vi "Find Multiple Items.vi"(7 "$Path or Item Name":string, 8 "error in (no error)":errorcluster, 10 "Offset":i32, 11 "JSON":string) -> (0 "error out":errorcluster, 1 "<JSON>":string[](array[string]) caption="<JSON>Items", 2 "Item Offsets":i32[](array[numeric]), 3 "Item Names":string[](array[string]))   [LabVIEW 2019, in "JSONtext.lvlib"]
doc: "Find the JSON items at the JSON Path specified and returns them as an array.\n\nPaths specify an item in a tree of nested Elements, and start with $. Each element is either in the form .name, for Object items, or [n] for Array index ([*] for all elements). Multiple Object items can be specified by the list form .[abc,def].\n\nIf the Path input does not start with a $, then it is interpreted as a single Object Item name, rather than a path.\n\nExample JSON:\n{\"A\":[{\"C\":123,\"D\":4},{\"C\":567,\"D\":8}],\"B\":{\"F\":9},\"E\":true}\nAt path $.A[*].C are 123 and 567\nAt path $.B (or just B) is {\"F\":9}\nAt path $.B.F is 9\nAt path $.[B,E] are {\"F\":9} and true"
uses:
  JSONtext.lvlib
  support/Unescape JSON string.vi
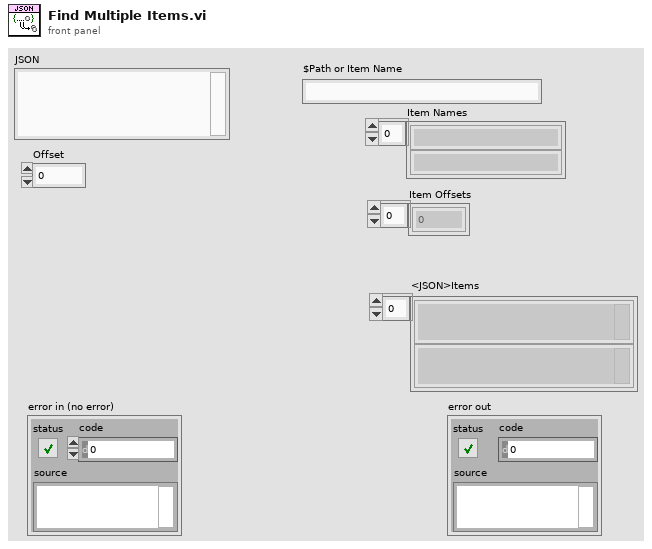
[diagram p1: front panel]
types:
  T1 = typedef "JSONtext.lvlib/Found Items.ctl" = cluster{"Item offset":i32, "Offset past Item":i32, "Name offset":i32, "Offset past Name":i32, "Found":bool, "Item Type":T2, "Item Index":i32, "Start Offset":i32, "Comma Needed For Insert":bool}
  T2 = typedef "JSONtext.lvlib/Parsing State.ctl" = enum16{"Parser Error", "Object", "Array", "String", "Number/Other", "Leading Whitespace", "Object end", "Array end", "Value end"}
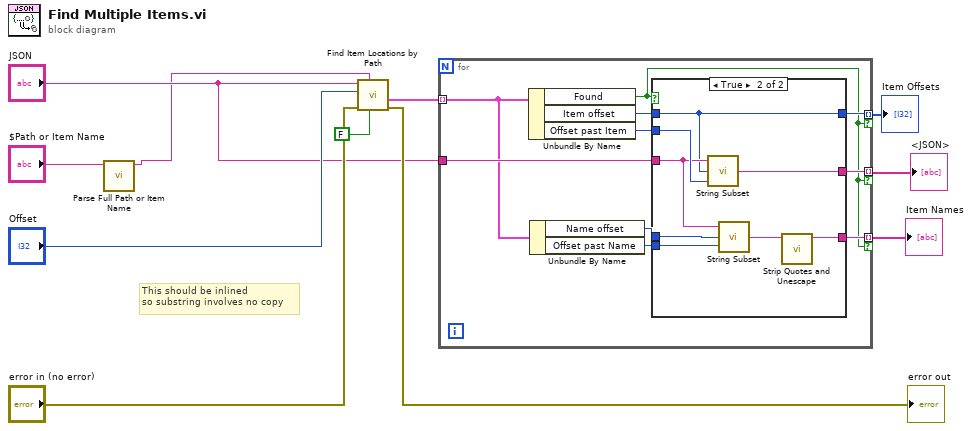
[diagram p0: block diagram]
diagram:
  # "This should be inlined\nso substring involves no copy"
  n1 = call "Parse Full Path or Item Name.vi"("Full Path (with $) or Name"="$Path or Item Name") -> ("Relative Path or JSON-format name"=w1:string)  [unwired: 10 in]
  n2 = call "Find Item Locations by Path.vi"("Only return first found"=FALSE, "Path"=w1, "error in (no error)"="error in (no error)", "Offset"="Offset", "JSON"="JSON") -> ("error out"=→"error out":errorcluster, "Items"=w6:T1[])  [unwired: 5 in]
  n3 = for {
    tunnel: "JSON" -> [w21]
    tunnel: [w20] -> w7 mode=indexing if=w12
    tunnel: w6 -> [w17] mode=indexing
    tunnel: [w14] -> w5 mode=indexing if=w12
    tunnel: [w13] -> w3 mode=indexing if=w12
    n4 = Unbundle By Name(w17) -> ("Found"=w12:bool, "Item offset"=w19:i32, "Offset past Item"=w18:i32)
    n5 = Unbundle By Name(w17) -> ("Name offset"=w15:i32, "Offset past Name"=w16:i32)
    n6 = case shown="True" w12 {
      tunnel: w21 -> [_ w27]
      tunnel: [_ w29] -> w20
      tunnel: w19 -> [_ w22]
      tunnel: w18 -> [_ w28]
      tunnel: w16 -> [_ w26]
      tunnel: w15 -> [_ w25]
      tunnel: [_ w23] -> w14
      tunnel: [_ w22] -> w13
      frame False {
      }
      frame True {
        n7 = call "String Subset.vi"("Offset past End"=w28, "Start offset"=w22, "JSON"=w27) -> ("substring"=w29:string)  [unwired: 2 in]
        n8 = call "String Subset.vi"("Offset past End"=w26, "Start offset"=w25, "JSON"=w27) -> ("substring"=w24:string)  [unwired: 2 in]
        n9 = call "Strip Quotes and Unescape.vi"("String"=w24) -> ("result string"=w23:string)  [unwired: 9 in, 1 out]
      }
    }
  }
  "<JSON>" <- w7
  "Item Names" <- w5
  "Item Offsets" <- w3
